vi "Set TDMS Channel Names.vi"(10 "Channel Names":string[](array[string]), 11 "App Data In":T1) -> (3 "App Data Out":T1)   [LabVIEW 2019]
uses:
  TypeDef/App Data.ctl
  TypeDef/File Type.ctl
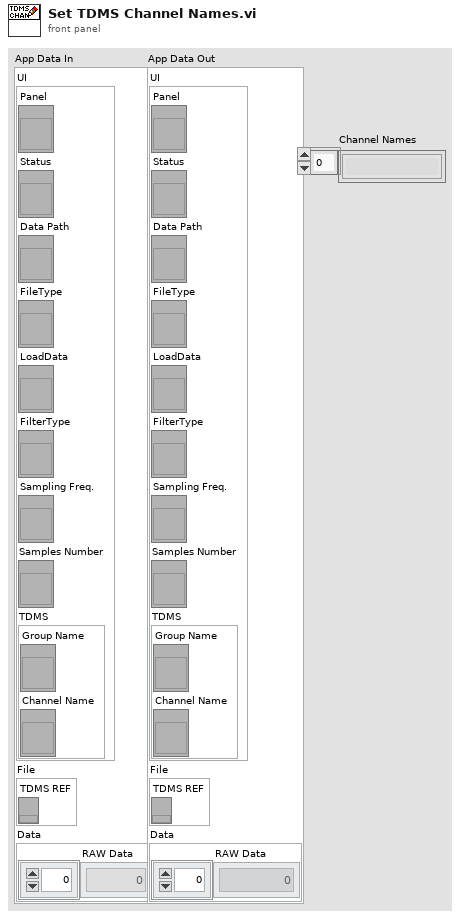
[diagram p1: front panel]
types:
  T1 = typedef "App Data.ctl" = cluster{"UI":cluster{"Panel":refnum<vi>, "Status":refnum<vi>, "Data Path":refnum<vi>, "FileType":refnum<vi>, "LoadData":refnum<vi>, "FilterType":refnum<vi>, "Sampling Freq.":refnum<vi>, "Samples Number":refnum<vi>, "TDMS":cluster{"Group Name":refnum<vi>, "Channel Name":refnum<vi>}}, "File":cluster{"TDMS REF":refnum<k34>}, "Data":cluster{"RAW Data":dbl[]}}
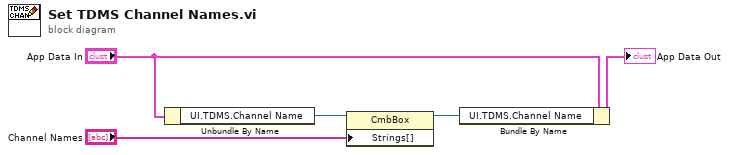
[diagram p0: block diagram]
diagram:
  n1 = Unbundle By Name("App Data In") -> ("UI.TDMS.Channel Name"=w4:refnum<vi>)
  n2 = property class="CmbBox"(reference=w4, "Strings[]"="Channel Names") -> (reference out=w5:refnum<vi>)  [unwired: 1 in, 1 out]
  n3 = Bundle By Name(cluster="App Data In", "UI.TDMS.Channel Name"=w5) -> (→"App Data Out":T1)
